vi "TDS Digital Input Multiple Read.vi"(8 "error in (no error)":errorcluster, 10 "Signal InstConfig":string, 11 "Address":string) -> (0 "error out":errorcluster, 3 "Input States":bool[](array[boolean]))   [LabVIEW 2025, in "Interface Functions.lvlib"]
uses:
  Interface Functions.lvlib
panel:
  # "Digital Input Multiple Read"
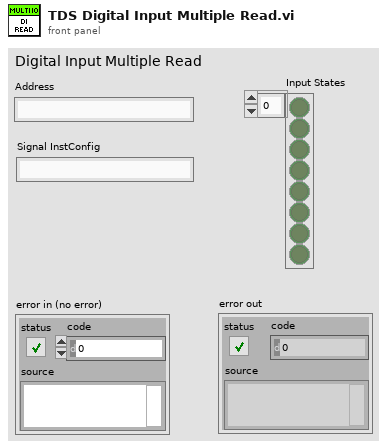
[diagram p1: front panel]
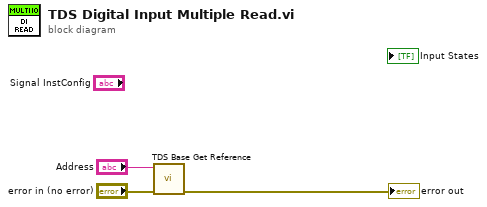
[diagram p0: block diagram]
diagram:
  n1 = call "TDS Base Get Reference.vi"("error in (no error)"="error in (no error)", "Address"="Address") -> ("error out"=→"error out":errorcluster)  [unwired: 8 in, 1 out]
